vi "PSDATA_Variant To Str.vi"(9 "error in":errorcluster, 10 "Value":variant) -> (1 "error out":errorcluster, 2 "Value":string, 4 "Str":string)   [LabVIEW 2016]
doc: "Developer：YDX"
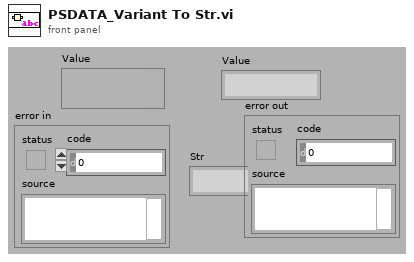
[diagram p1: front panel]
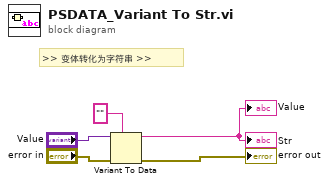
[diagram p0: block diagram]
diagram:
  # ">> 变体转化为字符串 >>"
  n1 = Variant To Data(error in="error in", type="" ("Str"), Variant="Value") -> (data=→"Value" →"Str":string, error out=→"error out":errorcluster)
